vi "Gabor Transform and Expansion.vi"() -> ()   [LabVIEW 2023]
doc: "This example shows how to use the TFA Discrete Gabor Transform VI and the TFA Discrete Gabor Expansion VI.\n\n<b>Instructions:</b>\n1) Run this VI.\n2) Compare the original signal and reconstructed signal.\n3) Browse the Block Diagram to learn how to use TFA Discrete Gabor Transform VI and the TFA Discrete Gabor Expansion VI with Dual Window Express VI."
uses:
  Instance           8 37Saved   Gabor Transform and Expansion .vi
  <vilib>/addons/Time Frequency Analysis/Transform.llb/TFA Discrete Gabor Transform (Waveform).vi
  <vilib>/addons/Time Frequency Analysis/Transform.llb/TFA Discrete Gabor Expansion (Waveform).vi
  <vilib>/addons/_Advanced Signal Processing/NI_AdvSigProcTFA.lvlib
  <vilib>/Analysis/NI_AALPro.lvlib
panel:
  in  "Data":u16(ring) items=["PC Fan"=0, "Noisy Chirps"=1, "TDR 1"=2, "TDR 2"=3, "Liquefaction"=4, "Liquefaction Free"=5, "Aneurysm"=6, "Bat"=7, "RF"=8, "Two Gaussian"=9, "Three Gaussian"=10, "Chirp"=11, "Gaussian Chirp"=12, "Cross Chirp"=13, "Doppler"=14, "HOP"=15, "TF Sine"=16, "Three Tone"=17, "Four Tone"=23, "Blood Flow Doppler (phase a)"=20, "Blood Flow Doppler (phase b)"=21, "Heart sound"=22, "Random Noise"=19]
  out "aspt-left-top":bool
  out "MSE":dbl format="%.1e"
  out "Magnitude of Gabor Coefficients":dbl[][](graph)
  out "Signals":waveform(dbl)[](graph)
  # "Overview: Shows how to use the TFA Discrete Gabor Transform VI and the TFA Discrete Gabor Expansion VI.\nRequirements: LabVIEW Full Development System, Advanced Signal Processing Toolkit\nInstructions: \n1. Run this VI.\n2. Compare the original signal and reconstructed signal.\n3. Browse the block diagram to learn how to use TFA Discrete Gabor Transform VI and the TFA Discrete Gabor Expansion VI with Dual Window Express VI."
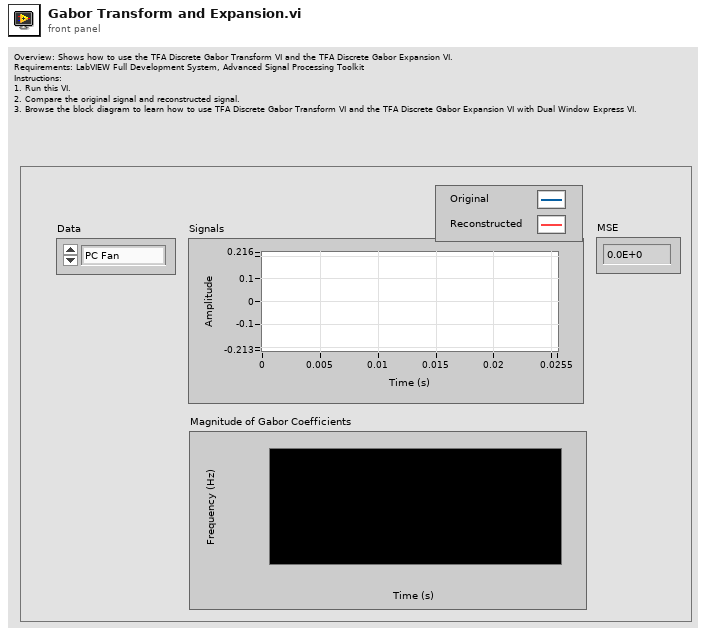
[diagram p1: front panel]
types:
  T1 = cluster{"synthesis window":dbl[], "dM (time steps)":i32, "N (frequency bins)":i32}
  T2 = cluster{"analysis window":dbl[], "dM (time steps)":i32, "N (frequency bins)":i32}
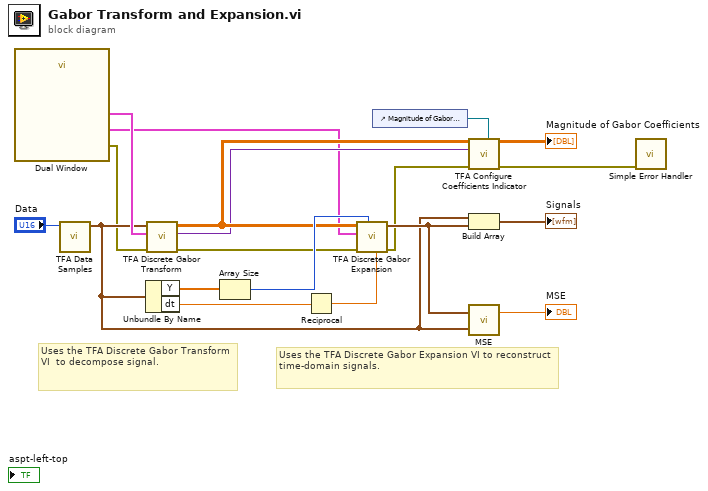
[diagram p0: block diagram]
diagram:
  # "Uses the TFA Discrete Gabor Expansion VI to reconstruct time-domain signals."
  # "Uses the TFA Discrete Gabor Transform VI  to decompose signal."
  n1 = call "Dual Window"() -> ("error out"=w1:errorcluster, "expansion info"=w9:T1, "transform info"=w10:T2)  [unwired: 1 in, 8 out]
  n2 = call <vilib>:"TFA Data Samples.vi"("data"="Data") -> ("signal"=w6:waveform(dbl))  [unwired: 10 out]
  n3 = Unbundle By Name(w6) -> ("Y"=w15:dbl[], "dt"=w18:dbl)
  n4 = call-poly <vilib>:"TFA Discrete Gabor Transform.vi"("error in (no error)"=w1, "transform info"=w10, "signal"=w6) -> ("error out"=w4:errorcluster, "scale info"=w13:variant, "Gabor coef"=w14:cdb[][])  [unwired: 6 out]
  n5 = Array Size(array=w15) -> (size(s)=w19:i32)
  n6 = Reciprocal(x=w18) -> (1/x=w17:dbl)
  n7 = call-poly <vilib>:"TFA Discrete Gabor Expansion.vi"("sampling rate"=w17, "signal length"=w19, "error in (no error)"=w4, "expansion info"=w9, "Gabor coef"=w14) -> ("error out"=w3:errorcluster, "signal"=w7:waveform(dbl))  [unwired: 5 out]
  n8 = control-ref of="Magnitude of Gabor Coefficients"() -> (w11:refnum<vi>)
  n9 = call <vilib>:"TFA Configure Coefficients Indicator.vi"("reference of TF coefficients indicator"=w11, "error in (no error)"=w3, "scale info"=w13, "TF coefficients"=w14) -> ("error out"=w2:errorcluster, "TF coefficients indicator"=→"Magnitude of Gabor Coefficients":dbl[][])  [unwired: 3 in, 3 out]
  n10 = Build Array(w6, w7) -> (→"Signals":waveform(dbl)[])
  n11 = call <vilib>:"MSE.vi"("X Values"=w6, "Y Values"=w7) -> ("mse"=→"MSE":dbl)  [unwired: 1 out]
  n12 = call <vilib>:"Simple Error Handler.vi"("error in (no error)"=w2) -> ()  [unwired: 4 in, 5 out]
